vi "config reader.vi"(0 "file path (use dialog)":path=path "S:/Students/Carl Camp/New Text Document.txt", 1 "error input":errorcluster) -> (2 "output array":string[](array[string]), 3 "x+y":i32, 4 "error output":errorcluster)   [LabVIEW 2012]
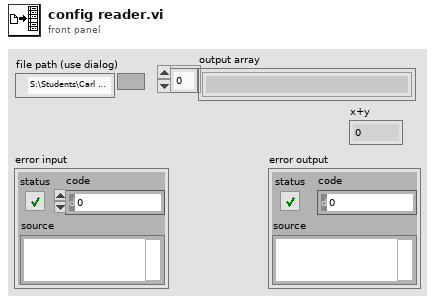
[diagram p1: front panel]
types:
  T1 = enum16{"open", "replace", "create", "open or create", "replace or create", "replace or create with confirmation"}
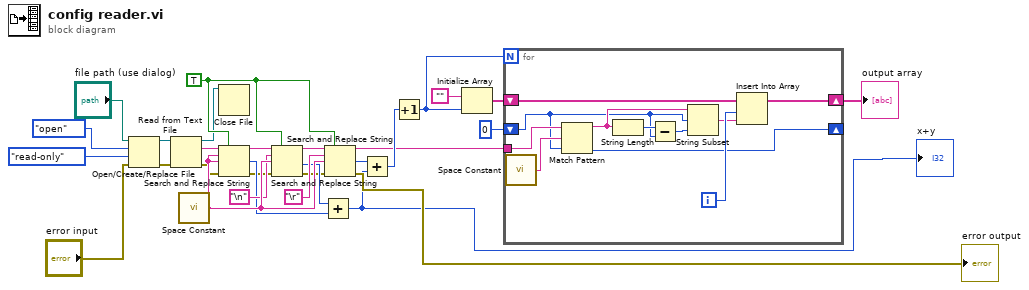
[diagram p0: block diagram]
diagram:
  w27 = TRUE ("replace all? (F)")
  n1 = Open/Create/Replace File(file path (use dialog)="file path (use dialog)", error in="error input", operation (0:open)=T1."open", access (0:read/write)=enum16{"read/write", "read-only", "write-only"}."read-only") -> (refnum out=w14:refnum<file>, error out=w3:errorcluster)  [unwired: 2 in, 1 out]
  n2 = Read from Text File(file (use dialog)=w14, error in=w3) -> (refnum out=w15:refnum<file>, text=w16:string, error out=w4:errorcluster)  [unwired: 2 in, 1 out]
  n3 = call <vilib>:"Space Constant.vi"() -> ("String"=w25:string)
  n4 = Close File(refnum=w15) -> ()  [unwired: 1 in, 2 out]
  n5 = Search and Replace String(replace all?=w27, input string=w16, search string=w25, replace string=w25, error in=w4) -> (result string=w9:string, number of replacements=w11:i32, error out=w5:errorcluster)  [unwired: 3 in, 1 out]
  n6 = Search and Replace String(replace all?=w27, input string=w9, search string="\n", replace string=w25, error in=w5) -> (result string=w22:string, number of replacements=w10:i32, error out=w6:errorcluster)  [unwired: 3 in, 1 out]
  n7 = Add(x=w10, y=w11) -> (x+y=w1:i32)
  "x+y" <- w1
  n8 = Search and Replace String(replace all?=w27, input string=w22, search string="\r", replace string=w25, error in=w6) -> (result string=w21:string, number of replacements=w23:i32, error out=→"error output":errorcluster)  [unwired: 3 in, 1 out]
  n9 = Add(x=w23, y=w1) -> (x+y=w24:i32)
  n10 = Increment(x=w24) -> (x+1=w28:i32)
  n11 = Initialize Array("", w28) -> (w19:string[])
  n12 = for {
    N: w28 -> [_]
    tunnel: w21 -> [w35]
    shift-right: [w39] -> w20
    shift-left: w19 -> [w40]
    shift-right: [w32] -> _
    shift-left: 0 ("offset past match") -> [w30]
    i -> [w38]
    n13 = call <vilib>:"Space Constant.vi"() -> ("String"=w36:string)
    n14 = Match Pattern(string=w35, regular expression=w36, offset (0)=w30) -> (before substring=w34:string, offset past match=w32:i32)  [unwired: 2 out]
    n15 = String Length(string=w34) -> (length=w31:i32)
    n16 = Subtract(x=w31, y=w30) -> (x-y=w33:i32)
    n17 = String Subset(string=w34, offset (0)=w30, length (rest)=w33) -> (substring=w37:string)
    n18 = Insert Into Array(array=w40, index=w38, new element=w37) -> (w39:string[])
  }
  "output array" <- w20
